vi "CCD3000 Pixel to Wavelength v10.0.0.vi"(2 "Wavelengths (nm)":dbl[](array[numeric]), 3 "Raw Spectrum":dbl[](array[numeric])) -> (0 "Spectrum-Array":dbl[][](array[numeric]), 1 "Spectrum-Cluster":T1)   [LabVIEW 2010]
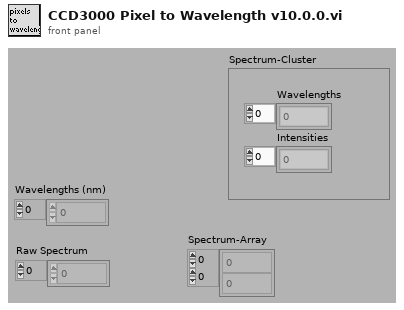
[diagram p1: front panel]
types:
  T1 = cluster{"Intensities":dbl[], "Wavelengths":dbl[]}
  T2 = cluster{"Wavelengths (nm)":dbl[], "Raw Spectrum":dbl[]}
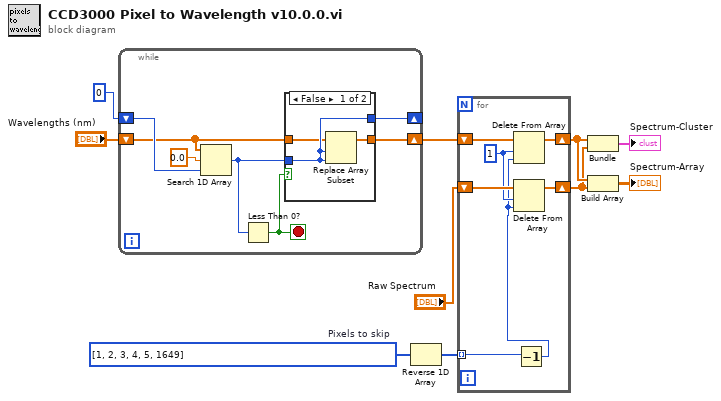
[diagram p0: block diagram]
diagram:
  w9 = i32[] [1, 2, 3, 4, 5, 1649]  # Pixels to skip
  n1 = while {
    shift-right: [w11] -> w3
    shift-left: "Wavelengths (nm)" -> [w14]
    shift-right: [w15] -> _
    shift-left: 0 ("index of element") -> [w16]
    stop <- w13 stop-if-true
    n2 = Search 1D Array(1D array=w14, element=0.0, start index (0)=w16) -> (index of element=w12:i32)
    n3 = Less Than 0?(x=w12) -> (x < 0?=w13:bool)
    n4 = case shown="False" w13 {
      tunnel: w12 -> [w20 w22]
      tunnel: [w20 w22] -> w15
      tunnel: w14 -> [w19 w21]
      tunnel: [w18 w21] -> w11
      frame False {
        n5 = Replace Array Subset(array=w19, new element=w20, index=w20) -> (w18:dbl[])
      }
      frame True {
      }
    }
  }
  n6 = Reverse 1D Array(array=w9) -> (reversed array=w1:i32[])
  n7 = for {
    shift-right: [w28] -> w8
    shift-left: w3 -> [w27]
    shift-right: [w29] -> w7
    shift-left: "Raw Spectrum" -> [w26]
    tunnel: w1 -> [w24] mode=indexing
    w25 = 1 ("length")
    n8 = Decrement(x=w24) -> (x-1=w23:i32)
    n9 = Delete From Array(array=w27, length=w25, index=w23) -> (array with subset deleted=w28:dbl[])  [unwired: 1 out]
    n10 = Delete From Array(array=w26, length=w25, index=w23) -> (array with subset deleted=w29:dbl[])  [unwired: 1 out]
  }
  n11 = Bundle("Wavelengths (nm)"=w8, "Raw Spectrum"=w7) -> (→"Spectrum-Cluster":T2)  [unwired: 1 in]
  n12 = Build Array(w8, w7) -> (→"Spectrum-Array":dbl[][])
